vi "Mouse Capture.vi"(8 "error in (no error)":errorcluster, 11 "ColorSelector in":refnum<class "ColorSelector.lvclass">) -> (0 "error out":errorcluster, 3 "ColorSelector (dup)":refnum<class "ColorSelector.lvclass">)   [LabVIEW 2015, in "ColorSelector.lvclass"]
doc: "This VI is launched asynchronously when the Grey or Color Selectors are clicked on. Its purpose is to capture the mouse move event everywhere on the screen or screens, send the coordinates back to the Event Handler, and close when a mouse up occurs.\n<b> </b> <b> </b>\n©2017 Q Software Innovations, LLC (QSI)\nwritten by Quentin Alldredge\nproduced in LabVIEW 2015\n\nsupport@qsoftwareinnovations.com\nwww.qsoftwareinnovations.com\n\nAll rights reserved.\n\nRedistribution and use in source and binary forms, with or without modification, are permitted provided that the following conditions are met:\n\n * Redistributions of source code must retain the above copyright notice, this list of conditions and the following disclaimer.\n * Redistributions in binary form must reproduce the above copyright notice, this list of conditions and the following disclaimer in the documentation and/or other materials provided with the distribution.\n * Neither the name of Q Software Innovations, LLC. nor the names of its contributors may be used to endorse or promote products derived from this software without specific prior written permission.\n\nTHIS SOFTWARE IS PROVIDED BY THE COPYRIGHT HOLDERS AND CONTRIBUTORS \"AS IS\" AND ANY EXPRESS OR IMPLIED WARRANTIES, INCLUDING, BUT NOT LIMITED TO, THE IMPLIED WARRANTIES OF MERCHANTABILITY AND FITNESS FOR A PARTICULAR PURPOSE ARE DISCLAIMED. IN NO EVENT SHALL THE COPYRIGHT OWNER OR CONTRIBUTORS BE LIABLE FOR ANY DIRECT, INDIRECT, INCIDENTAL, SPECIAL, EXEMPLARY, OR CONSEQUENTIAL DAMAGES (INCLUDING, BUT NOT LIMITED TO, PROCUREMENT OF SUBSTITUTE GOODS OR SERVICES; LOSS OF USE, DATA, OR PROFITS; OR BUSINESS INTERRUPTION) HOWEVER CAUSED AND ON ANY THEORY OF LIABILITY, WHETHER IN CONTRACT, STRICT LIABILITY, OR TORT (INCLUDING NEGLIGENCE OR OTHERWISE) ARISING IN ANY WAY OUT OF THE USE OF THIS SOFTWARE, EVEN IF ADVISED OF THE POSSIBILITY OF SUCH DAMAGE."
uses:
  ColorSelector.lvclass
  ColorSelector.lvclass/ColorSelector.ctl
  <vilib>/Utility/miscctls.llb/LVRectTypeDef.ctl
types:
  T1 = enum32{"Invalid", "Standard", "Closed", "Hidden", "Minimized", "Maximized"}
  T2 = typedef "LVRectTypeDef.ctl" = cluster{"Left":i16, "Top":i16, "Right":i16, "Bottom":i16}
  T3 = typedef "LVAllMonitorsDisplayTypeDef.ctl" = cluster{"Bounds":cluster{"Left":i16, "Top":i16, "Right":i16, "Bottom":i16}, "Depth":i16}[]
  T4 = cluster{"Left":i32, "Top":i32, "Right":i32, "Bottom":i32}
  T5 = typedef "LVPoint32TypeDef.ctl" = cluster{"Horizontal":i32, "Vertical":i32}
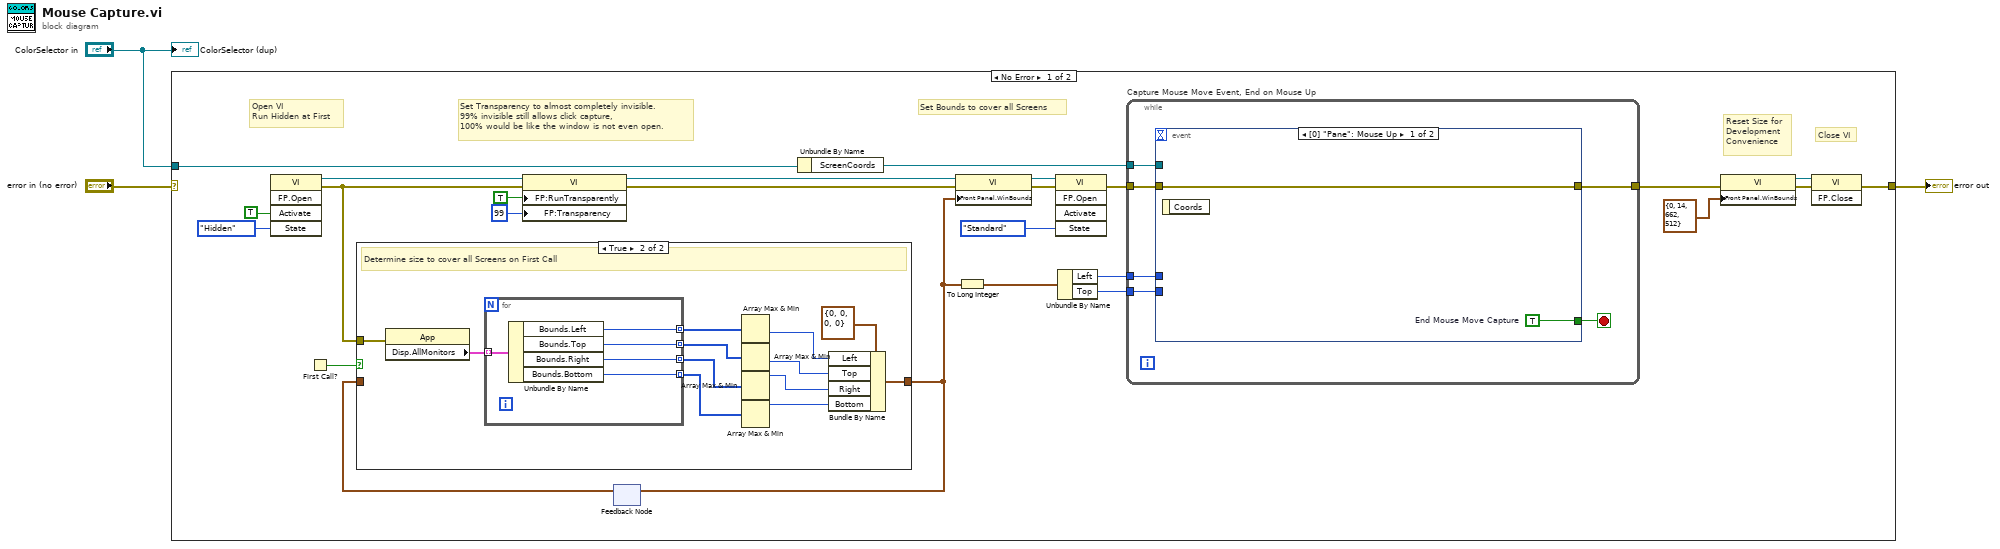
[diagram p0: block diagram]
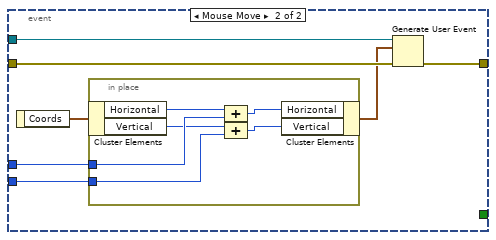
[diagram p3: hidden frame]
diagram:
  n1 = case shown="No Error" "error in (no error)" {
    selector: "error in (no error)" -> [_ w68]
    tunnel: [w11 w68] -> w2
    tunnel: "ColorSelector in" -> [w15 _]
    frame No Error {
      # "Close VI"
      # "Reset Size for \nDevelopment\nConvenience"
      # "Set Transparency to almost completely invisible.  \n99% invisible still allows click capture, \n100% would be like the window is not even open."
      # "Open VI\nRun Hidden at First"
      # "Set Bounds to cover all Screens"
      n2 = invoke class="VI" method="FP.Open"("Activate"=TRUE ("Activate?"), "State"=T1."Hidden") -> (reference out=w24:refnum<vi>, error out=w8:errorcluster)  [unwired: 3 in, 3 out]
      n3 = First Call?() -> (First Call?: T/F=w10:bool)
      n4 = property class="VI"(reference=w24, error in=w8, "FP:RunTransparently"=TRUE ("Front Panel Window:Run VI Transparently"), "FP:Transparency"=u8 99 ("Front Panel Window:Transparency")) -> (reference out=w23:refnum<vi>, error out=w16:errorcluster)
      n5 = feedback #1() -> (w9:T2)  [unwired: 1 in]
      n6 = case shown="True" w10 {
        tunnel: [w29 w33] -> w7
        tunnel: w8 -> [_ w30]
        tunnel: w9 -> [w29 _]
        frame False {
          # "Get Screen Bounds from Feedback Node Functional Global Variable"
        }
        frame True {
          # "Determine size to cover all Screens on First Call"
          n7 = property class="App"(error in=w30) -> ("Disp.AllMonitors"=w41:T3)  [unwired: 1 in, 2 out]
          n8 = for {
            tunnel: w41 -> [w46] mode=indexing
            tunnel: [w45] -> w40 mode=indexing
            tunnel: [w44] -> w39 mode=indexing
            tunnel: [w43] -> w38 mode=indexing
            tunnel: [w42] -> w37 mode=indexing
            n9 = Unbundle By Name(w46) -> ("Bounds.Left"=w45:i16, "Bounds.Top"=w44:i16, "Bounds.Right"=w43:i16, "Bounds.Bottom"=w42:i16)
          }
          n10 = Array Max & Min(array=w40) -> (min value=w35:i16)  [unwired: 3 out]
          n11 = Array Max & Min(array=w39) -> (min value=w31:i16)  [unwired: 3 out]
          n12 = Array Max & Min(array=w38) -> (max value=w32:i16)  [unwired: 3 out]
          n13 = Array Max & Min(array=w37) -> (max value=w34:i16)  [unwired: 3 out]
          n14 = Bundle By Name(cluster=T2 {"Left"=0, "Top"=0, "Right"=0, "Bottom"=0} ("Front Panel Window:Window Bounds"), "Left"=w35, "Top"=w31, "Right"=w32, "Bottom"=w34) -> (w33:T2)
        }
      }
      n15 = feedback-in #1(w7) -> ()
      n16 = Unbundle By Name(w15) -> ("ScreenCoords"=w14:refnum<user-event>)
      n17 = property class="VI"(reference=w23, error in=w16, "Front Panel.WinBounds"=w7) -> (reference out=w20:refnum<vi>, error out=w22:errorcluster)
      n18 = To Long Integer(number=w7) -> (32bit integer=w5:T4)
      n19 = invoke class="VI" method="FP.Open"(reference=w20, error in=w22, "State"=T1."Standard") -> (error out=w21:errorcluster)  [unwired: 2 in, 4 out]
      n20 = Unbundle By Name(w5) -> ("Left"=w6:i32, "Top"=w4:i32)
      n21 = while "Capture Mouse Move Event, End on Mouse Up" {
        tunnel: w21 -> [w52]
        tunnel: [w51] -> w28
        tunnel: w14 -> [w49]
        tunnel: w6 -> [w48]
        tunnel: w4 -> [w47]
        stop <- w50 stop-if-true
        n22 = event shown="[0] \"Pane\": Mouse Up" {
          selector: _ -> [_ _]
          dyn-events: _ -> [_ _]
          timeout: _ -> [_ _]
          tunnel: w52 -> [w54 w59]
          tunnel: [w54 w60] -> w51
          tunnel: [w53 _] -> w50
          tunnel: w49 -> [_ w61]
          tunnel: w48 -> [_ w56]
          tunnel: w47 -> [_ w55]
          event Mouse Up {
            w53 = TRUE  # End Mouse Move Capture
            n23 = event-data() -> ()  [unwired: 1 in, 1 out]
          }
          event Mouse Move {
            n24 = event-data() -> ("Coords"=w58:T5)  [unwired: 1 in]
            n25 = in-place {
              in-place-border: w56 -> [w66]
              in-place-border: w55 -> [w64]
              n26 = in-place-cluster #2(w58) -> ("Horizontal"=w67:i32, "Vertical"=w65:i32)
              n27 = Compound Arithmetic op=ADD(w67, w66) -> (w63:i32)
              n28 = Compound Arithmetic op=ADD(w65, w64) -> (w62:i32)
              n29 = in-place-cluster #2("Horizontal"=w63, "Vertical"=w62) -> (w57:T5)
            }
            n30 = Generate User Event(user event=w61, event data cluster=w57, error in=w59) -> (error out=w60:errorcluster)  [unwired: 1 in, 1 out]
          }
        }
      }
      n31 = property class="VI"(error in=w28, "Front Panel.WinBounds"=T2 {"Left"=0, "Top"=14, "Right"=662, "Bottom"=512} ("Front Panel Window:Window Bounds")) -> (reference out=w13:refnum<vi>, error out=w12:errorcluster)  [unwired: 1 in]
      n32 = invoke class="VI" method="FP.Close"(reference=w13, error in=w12) -> (error out=w11:errorcluster)  [unwired: 1 in, 2 out]
    }
    frame Error {
    }
  }
  "error out" <- w2
  "ColorSelector (dup)" <- "ColorSelector in"
